vi "TCP-Quit Server (subnet).vi"(7 "Name":string, 9 "receiver port":u16=10000, 11 "error in (no error)":errorcluster) -> (15 "error out":errorcluster)   [LabVIEW 2020]
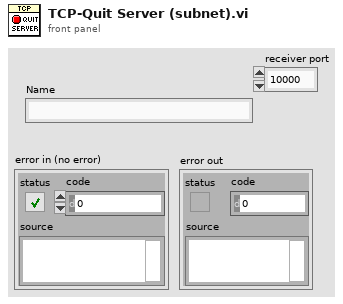
[diagram p1: front panel]
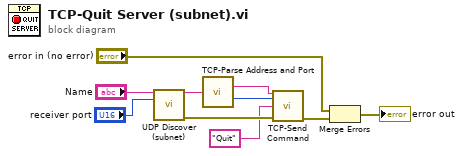
[diagram p0: block diagram]
diagram:
  n1 = call "UDP Discover (subnet).vi"("Name"="Name", "receiver port"="receiver port") -> ("address:port"=w6:string, "error out"=w10:errorcluster)  [unwired: 9 in, 3 out]
  n2 = call "TCP-Parse Address and Port.vi"("Address in"=w6) -> ("Address"=w5:string, "Port"=w4:i32)  [unwired: 12 in, 1 out]
  n3 = call "TCP-Send Command.vi"("PXI Address"=w5, "Port"=w4, "Command"="Quit", "error in (no error)"=w10) -> ("error out"=w7:errorcluster)  [unwired: 11 in]
  n4 = Merge Errors("error in (no error)", w7) -> (→"error out":errorcluster)
